vi "Diff_Drive_System_AutoTune_Dash_Write.vi"   [LabVIEW 2019]
uses:
  Diff_Drive_System_Globals.vi
  <vilib>/Rock Robotics/Network Tables/NT Write Boolean Array.vi
  <vilib>/Rock Robotics/WPI/ThirdParty/JAS_Junk/TrajLib/Trajectory_Library.lvlib
  <vilib>/Rock Robotics/Network Tables/NT Write Number.vi
  <vilib>/Rock Robotics/Network Tables/NT Write Numeric Array.vi
types:
  T1 = enum16{"Moving Average", "Low Pass 1st Order Butterworth", "Low Pass 2nd Order Butterworth", "High Pass 1st Order Butterworth", "High Pass 2nd Order Butterworth"}
  T2 = cluster{"proportional gain (Kp)":dbl, "integral time (Ki / Sec)":dbl, "derivative time (Kd /Sec)":dbl}
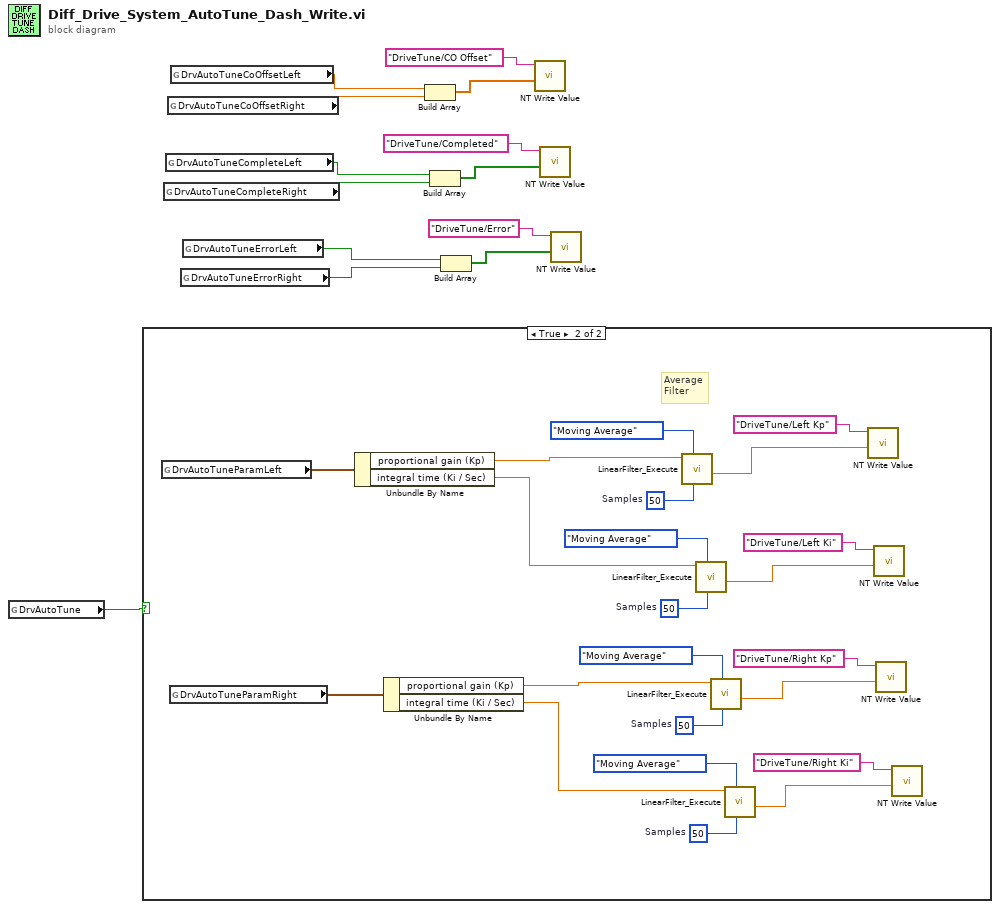
[diagram p0: block diagram]
diagram:
  n1 = global read "Diff_Drive_System_Globals.vi" "DrvAutoTune"() -> (w1:bool)
  n2 = case shown="True" w1 {
    frame False {
    }
    frame True {
      w24 = 50  # Samples
      w27 = 50  # Samples
      w30 = 50  # Samples
      w33 = 50  # Samples
      # "Average\nFilter"
      n3 = global read "Diff_Drive_System_Globals.vi" "DrvAutoTuneParamLeft"() -> (w34:T2)
      n4 = global read "Diff_Drive_System_Globals.vi" "DrvAutoTuneParamRight"() -> (w21:T2)
      n5 = Unbundle By Name(w34) -> ("proportional gain (Kp)"=w31:dbl, "integral time (Ki / Sec)"=w28:dbl)
      n6 = Unbundle By Name(w21) -> ("proportional gain (Kp)"=w25:dbl, "integral time (Ki / Sec)"=w22:dbl)
      n7 = call <vilib>:"LinearFilter_Execute.vi"("Samples"=w33, "Filter Type"=T1."Moving Average", "Input"=w31) -> ("Output"=w20:dbl)  [unwired: 7 in, 1 out]
      n8 = call <vilib>:"LinearFilter_Execute.vi"("Samples"=w30, "Filter Type"=T1."Moving Average", "Input"=w28) -> ("Output"=w14:dbl)  [unwired: 7 in, 1 out]
      n9 = call <vilib>:"LinearFilter_Execute.vi"("Samples"=w27, "Filter Type"=T1."Moving Average", "Input"=w25) -> ("Output"=w15:dbl)  [unwired: 7 in, 1 out]
      n10 = call <vilib>:"LinearFilter_Execute.vi"("Samples"=w24, "Filter Type"=T1."Moving Average", "Input"=w22) -> ("Output"=w16:dbl)  [unwired: 7 in, 1 out]
      n11 = call-poly <vilib>:"NT Write Value.vi"("Numeric"=w20, "Name"="DriveTune/Left Kp") -> ()  [unwired: 9 in, 1 out]
      n12 = call-poly <vilib>:"NT Write Value.vi"("Numeric"=w14, "Name"="DriveTune/Left Ki") -> ()  [unwired: 9 in, 1 out]
      n13 = call-poly <vilib>:"NT Write Value.vi"("Numeric"=w15, "Name"="DriveTune/Right Kp") -> ()  [unwired: 9 in, 1 out]
      n14 = call-poly <vilib>:"NT Write Value.vi"("Numeric"=w16, "Name"="DriveTune/Right Ki") -> ()  [unwired: 9 in, 1 out]
    }
  }
  n15 = global read "Diff_Drive_System_Globals.vi" "DrvAutoTuneCompleteRight"() -> (w4:bool)
  n16 = global read "Diff_Drive_System_Globals.vi" "DrvAutoTuneCompleteLeft"() -> (w5:bool)
  n17 = global read "Diff_Drive_System_Globals.vi" "DrvAutoTuneCoOffsetRight"() -> (w6:dbl)
  n18 = global read "Diff_Drive_System_Globals.vi" "DrvAutoTuneCoOffsetLeft"() -> (w7:dbl)
  n19 = global read "Diff_Drive_System_Globals.vi" "DrvAutoTuneErrorRight"() -> (w2:bool)
  n20 = global read "Diff_Drive_System_Globals.vi" "DrvAutoTuneErrorLeft"() -> (w3:bool)
  n21 = Build Array(w7, w6) -> (w8:dbl[])
  n22 = Build Array(w5, w4) -> (w10:bool[])
  n23 = Build Array(w3, w2) -> (w12:bool[])
  n24 = call-poly <vilib>:"NT Write Value.vi"("Numeric Array"=w8, "Name"="DriveTune/CO Offset") -> ()  [unwired: 9 in, 1 out]
  n25 = call-poly <vilib>:"NT Write Value.vi"("Boolean Array"=w10, "Name"="DriveTune/Completed") -> ()  [unwired: 9 in, 1 out]
  n26 = call-poly <vilib>:"NT Write Value.vi"("Boolean Array"=w12, "Name"="DriveTune/Error") -> ()  [unwired: 9 in, 1 out]
